vi "Accuracy_Calc.vi"() -> ()   [LabVIEW 2014]
uses:
  <vilib>/Utility/file.llb/Read From Spreadsheet File (string).vi
  <vilib>/Utility/file.llb/Write To Spreadsheet File (DBL).vi
panel:
  out "online_folder":string
  out "error out 2":errorcluster={"status"=TRUE, "code"=10, "source"="Create Folder in Trainging_Set_For_ LDA_Matrix_RSVP.vi<APPEND>\nC:\\Emotion_Research\\_Training_Test(LDA)\\2014-08-30"}
  out "error out":errorcluster={"status"=TRUE, "code"=10, "source"="Create Folder in Trainging_Set_For_ LDA_Matrix_RSVP.vi<APPEND>\nC:\\Emotion_Research\\_Training_Test(LDA)\\2014-08-30"}
  in  "피험자 이름":path
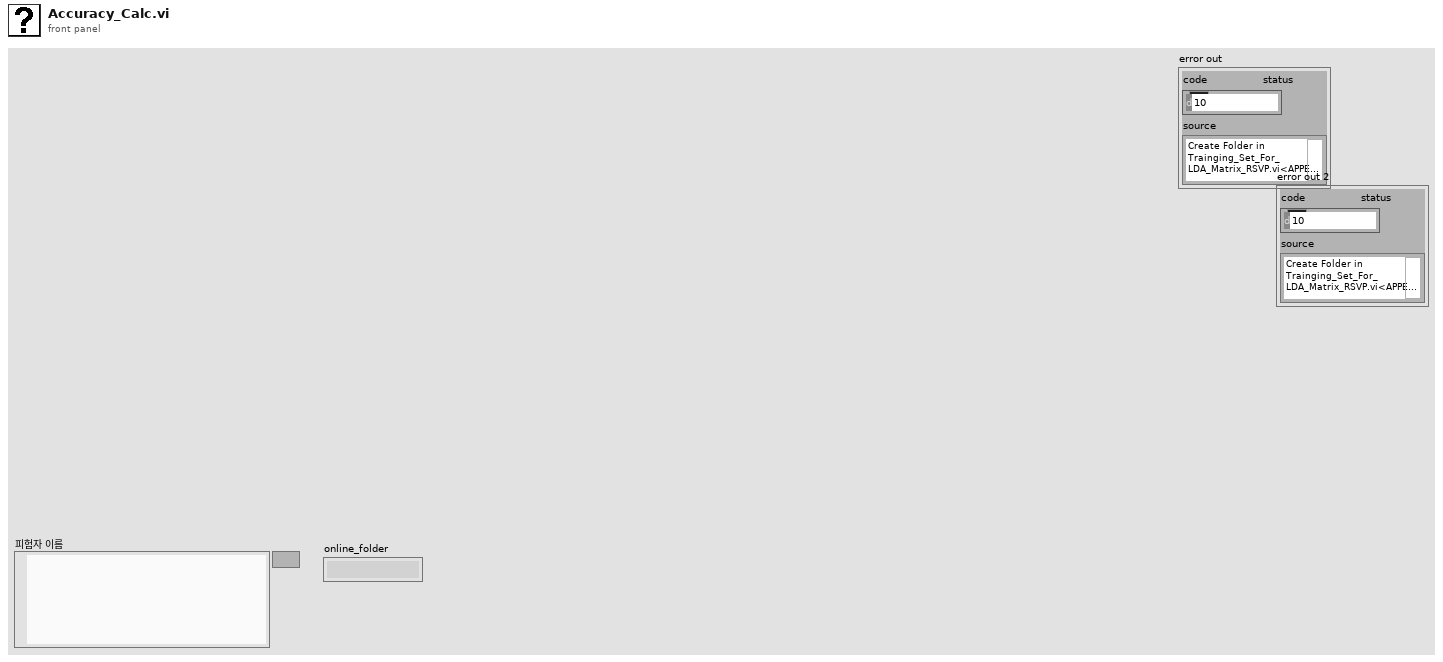
[diagram p1: front panel]
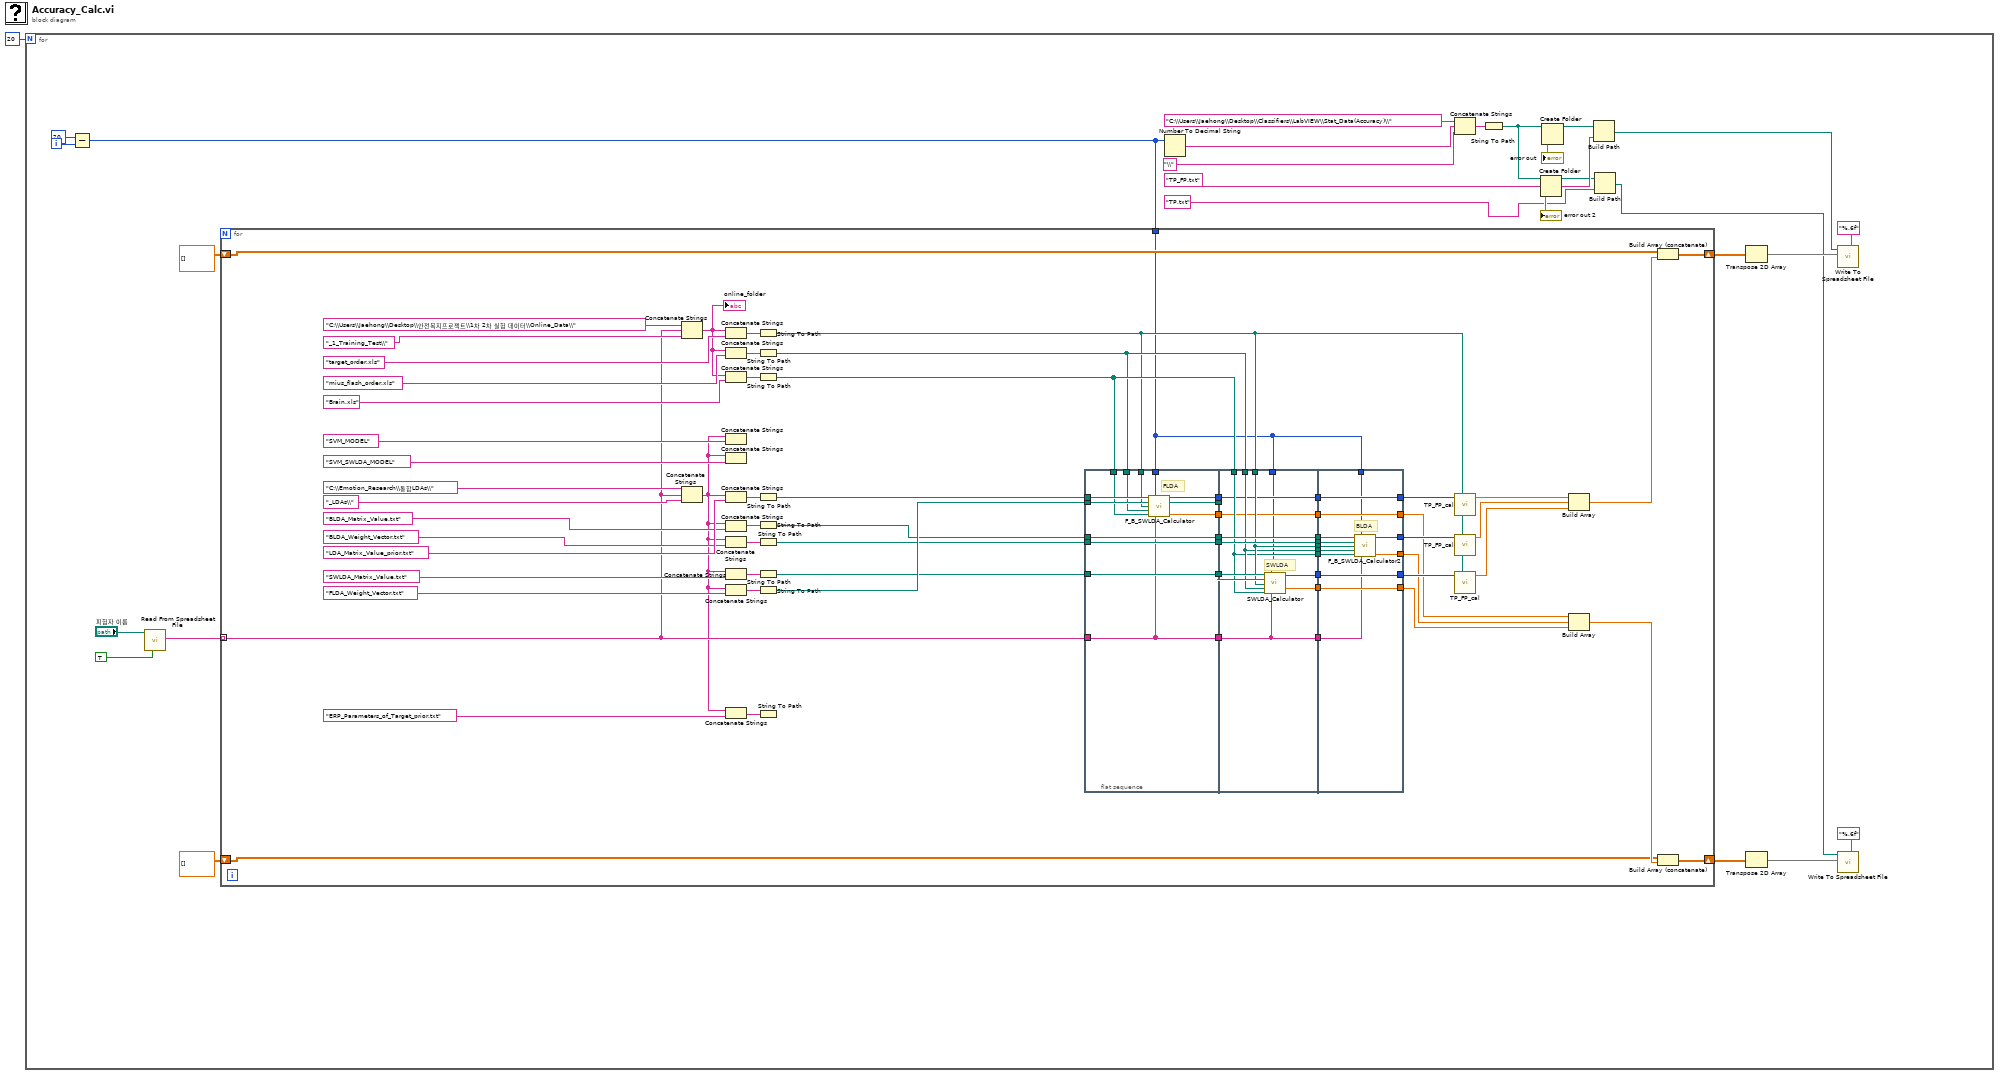
[diagram p0: block diagram]
diagram:
  n1 = for {
    N: 20 -> [_]
    i -> [w14]
    n2 = Subtract(x=20, y=w14) -> (x-y=w13:i32)
    n3 = call-poly <vilib>:"Read From Spreadsheet File.vi"("transpose (no:F)"=TRUE, "file path (dialog if empty)"="피험자 이름") -> ("first row"=w20:string[])  [unwired: 5 in, 4 out]
    n4 = for {
      shift-right: [w60] -> w26
      shift-left: dbl[][] [] -> [w59]
      shift-right: [w57] -> w24
      shift-left: dbl[][] [] -> [w56]
      tunnel: w20 -> [w55] mode=indexing
      tunnel: w13 -> [w30]
      n5 = Concatenate Strings("C:\\Users\\Jaehong\\Desktop\\안전복지프로젝트\\1차 2차 실험 데이터\\Online_Data\\", w55, "_1_Training_Test\\") -> (w69:string)
      "online_folder" <- w69
      n6 = Concatenate Strings("C:\\Emotion_Research\\통합LDAs\\", w55, "_LDAs\\") -> (w29:string)
      n7 = Concatenate Strings(w69, "target_order.xls") -> (w84:string)
      n8 = Concatenate Strings(w69, "mius_flash_order.xls") -> (w83:string)
      n9 = Concatenate Strings(w69, "Brain.xls") -> (w82:string)
      n10 = Concatenate Strings(w29, "SVM_MODEL") -> ()  [unwired: 1 out]
      n11 = Concatenate Strings(w29, "SVM_SWLDA_MODEL") -> ()  [unwired: 1 out]
      n12 = Concatenate Strings(w29, "LDA_Matrix_Value_prior.txt") -> (w94:string)
      n13 = Concatenate Strings(w29, "BLDA_Matrix_Value.txt") -> (w78:string)
      n14 = Concatenate Strings(w29, "BLDA_Weight_Vector.txt") -> (w77:string)
      n15 = Concatenate Strings(w29, "SWLDA_Matrix_Value.txt") -> (w80:string)
      n16 = Concatenate Strings(w29, "FLDA_Weight_Vector.txt") -> (w90:string)
      n17 = Concatenate Strings(w29, "ERP_Parameters_of_Target_prior.txt") -> (w72:string)
      n18 = String To Path(string=w84) -> (path=w37:path)
      n19 = String To Path(string=w83) -> (path=w38:path)
      n20 = String To Path(string=w82) -> (path=w39:path)
      n21 = String To Path(string=w94) -> (path=w91:path)
      n22 = String To Path(string=w78) -> (path=w75:path)
      n23 = String To Path(string=w77) -> (path=w76:path)
      n24 = String To Path(string=w80) -> (path=w67:path)
      n25 = String To Path(string=w90) -> (path=w81:path)
      n26 = String To Path(string=w72) -> ()  [unwired: 1 out]
      n27 = flat-sequence {
        tunnel: w55 -> [w100]
        tunnel: w67 -> [w106]
        tunnel: w75 -> [w107]
        tunnel: w76 -> [w108]
        tunnel: w81 -> [w104]
        tunnel: w91 -> [w105]
        tunnel: [w104] -> w44
        tunnel: [w108] -> w43
        tunnel: [w107] -> w42
        tunnel: [w106] -> w41
        tunnel: [w100] -> w40
        tunnel: w39 -> [w101]
        tunnel: w38 -> [w102]
        tunnel: w37 -> [w103]
        tunnel: [w99] -> w36
        tunnel: [w98] -> w33
        tunnel: w30 -> [w97]
        tunnel: w38 -> [w114]
        tunnel: w39 -> [w113]
        tunnel: w37 -> [w115]
        tunnel: [w119] -> w54
        tunnel: [w118] -> w53
        tunnel: [w117] -> w52
        tunnel: [w116] -> w51
        tunnel: [w115] -> w50
        tunnel: [w114] -> w49
        tunnel: [w113] -> w48
        tunnel: [w112] -> w47
        tunnel: w44 -> [w121]
        tunnel: w43 -> [w116]
        tunnel: w42 -> [w117]
        tunnel: w41 -> [w120]
        tunnel: w40 -> [w112]
        tunnel: w36 -> [w111]
        tunnel: [w111] -> w35
        tunnel: w33 -> [w110]
        tunnel: [w110] -> w32
        tunnel: w30 -> [w109]
        tunnel: [w133] -> w62
        tunnel: [w134] -> w66
        tunnel: w54 -> [w134]
        tunnel: w53 -> [w133]
        tunnel: w52 -> [w132]
        tunnel: w51 -> [w131]
        tunnel: w50 -> [w130]
        tunnel: w49 -> [w129]
        tunnel: w48 -> [w128]
        tunnel: w47 -> [w127]
        tunnel: [w126] -> w46
        tunnel: [w125] -> w45
        tunnel: w35 -> [w124]
        tunnel: [w124] -> w34
        tunnel: w32 -> [w123]
        tunnel: [w123] -> w31
        tunnel: w30 -> [w122]
        frame #0 {
          # "FLDA"
          n28 = call "F_B_SWLDA_Calculator.vi"("LDA_matrix"=w105, "Flash_Repeat"=w97, "Weight"=w104, "Target_order.txt"=w103, "mius_flash_order"=w102, "Brain"=w101, "피험자이름"=w100) -> ("ERP_발생_total"=w99:i16[], "ACC(%)"=w98:dbl)  [unwired: 7 in]
        }
        frame #1 {
          # "SWLDA"
          n29 = call "SWLDA_Calculator.vi"("LDA_matrix"=w120, "Flash_Repeat"=w109, "Weight"=w121, "Target_order.txt"=w115, "mius_flash_order"=w114, "Brain"=w113, "피험자이름"=w112) -> ("ERP_발생_total"=w119:i16[], "ACC(%)"=w118:dbl)  [unwired: 6 in, 1 out]
        }
        frame #2 {
          # "BLDA"
          n30 = call "F_B_SWLDA_Calculator2.vi"("LDA_matrix"=w132, "Flash_Repeat"=w122, "Weight"=w131, "Target_order.txt"=w130, "mius_flash_order"=w129, "Brain"=w128, "피험자이름"=w127) -> ("ERP_발생_total"=w126:i16[], "ACC(%)"=w125:dbl)  [unwired: 7 in]
        }
      }
      n31 = call "TP_FP_cal.vi"("Target_order"=w37, "ERP_발생_total"=w34) -> ("TP+FP(%)"=w65:dbl)  [unwired: 9 in]
      n32 = call "TP_FP_cal.vi"("Target_order"=w37, "ERP_발생_total"=w46) -> ("TP+FP(%)"=w64:dbl)  [unwired: 9 in]
      n33 = call "TP_FP_cal.vi"("Target_order"=w37, "ERP_발생_total"=w66) -> ("TP+FP(%)"=w63:dbl)  [unwired: 9 in]
      n34 = Build Array(w65, w64, w63) -> (w61:dbl[])
      n35 = Build Array(w31, w45, w62) -> (w58:dbl[])
      n36 = Build Array (concatenate)(w59, w61) -> (w60:dbl[][])
      n37 = Build Array (concatenate)(w56, w58) -> (w57:dbl[][])
    }
    n38 = Number To Decimal String(number=w13) -> (decimal integer string=w16:string)  [unwired: 1 in]
    n39 = Concatenate Strings("C:\\Users\\Jaehong\\Desktop\\Classifiers\\LabVIEW\\Stat_Data(Accuracy)\\", w16, "\\" ("string")) -> (w10:string)
    n40 = String To Path(string=w10) -> (path=w5:path)
    n41 = Create Folder(path (use dialog)=w5) -> (created path=w4:path, error out=→"error out 2":errorcluster)  [unwired: 2 in, 1 out]
    n42 = Create Folder(path (use dialog)=w5) -> (created path=w9:path, error out=→"error out":errorcluster)  [unwired: 2 in, 1 out]
    n43 = Build Path(base path=w9, name or relative path="TP_FP.txt") -> (appended path=w7:path)
    n44 = Build Path(base path=w4, name or relative path="TP.txt") -> (appended path=w2:path)
    n45 = Transpose 2D Array(2D array=w26) -> (transposed array=w19:dbl[][])
    n46 = Transpose 2D Array(2D array=w24) -> (transposed array=w18:dbl[][])
    n47 = call-poly <vilib>:"Write To Spreadsheet File.vi"("format (%.3f)"="%.6f", "2D data"=w19, "file path (dialog if empty)"=w7) -> ()  [unwired: 5 in, 1 out]
    n48 = call-poly <vilib>:"Write To Spreadsheet File.vi"("format (%.3f)"="%.6f", "2D data"=w18, "file path (dialog if empty)"=w2) -> ()  [unwired: 5 in, 1 out]
  }
